vi "ScaledInertialPropertiesToMJ.vi"() -> ()   [LabVIEW 2011]
uses:
  <vilib>/Utility/file.llb/Read From Spreadsheet File (DBL).vi
panel:
  out "pos values":dbl[](array[numeric])
  out "pos":string[](array[string])
  in  "template path":path=path "C:/Users/PPL/Documents/Visual Studio 2015/Projects/Mujoco/mjpro140/RMsimSibelius/5SegRM_template.xml"
  in  "RMsim path":path=path "C:/Users/PPL/Documents/Visual Studio 2015/Projects/Mujoco/mjpro140/RMsim"
  in  "SAVE":bool
  in  "RMsibelius path":path=path "C:/Users/PPL/Documents/Visual Studio 2015/Projects/Mujoco/mjpro140/RMsimSibelius"
  out "mass values":dbl[](array[numeric])
  out "masses":string[](array[string])
  out "length values":dbl[](array[numeric])
  out "lengths":string[](array[string])
  out "radii values":dbl[](array[numeric])
  out "radii":string[](array[string])
  out "MOI values":dbl[](array[numeric])
  out "appended array":string[](array[string])
  in  "indices":dbl[](array[numeric])=[0.0, 2.0, 3.0, 4.0, 5.0]
  in  "file path (dialog if empty)":path
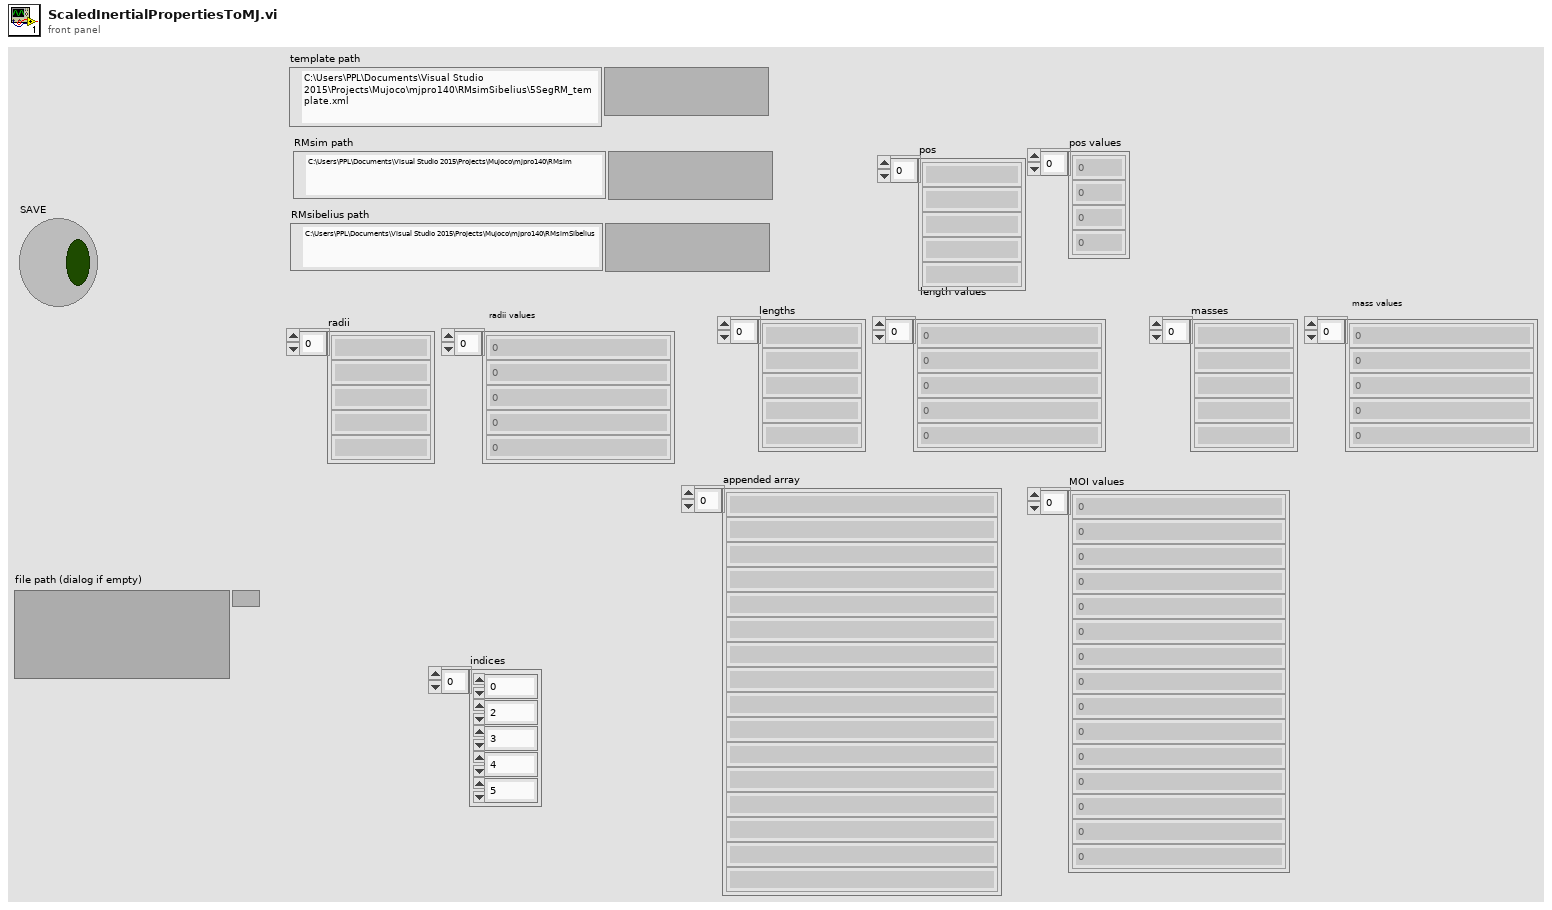
[diagram p1: front panel]
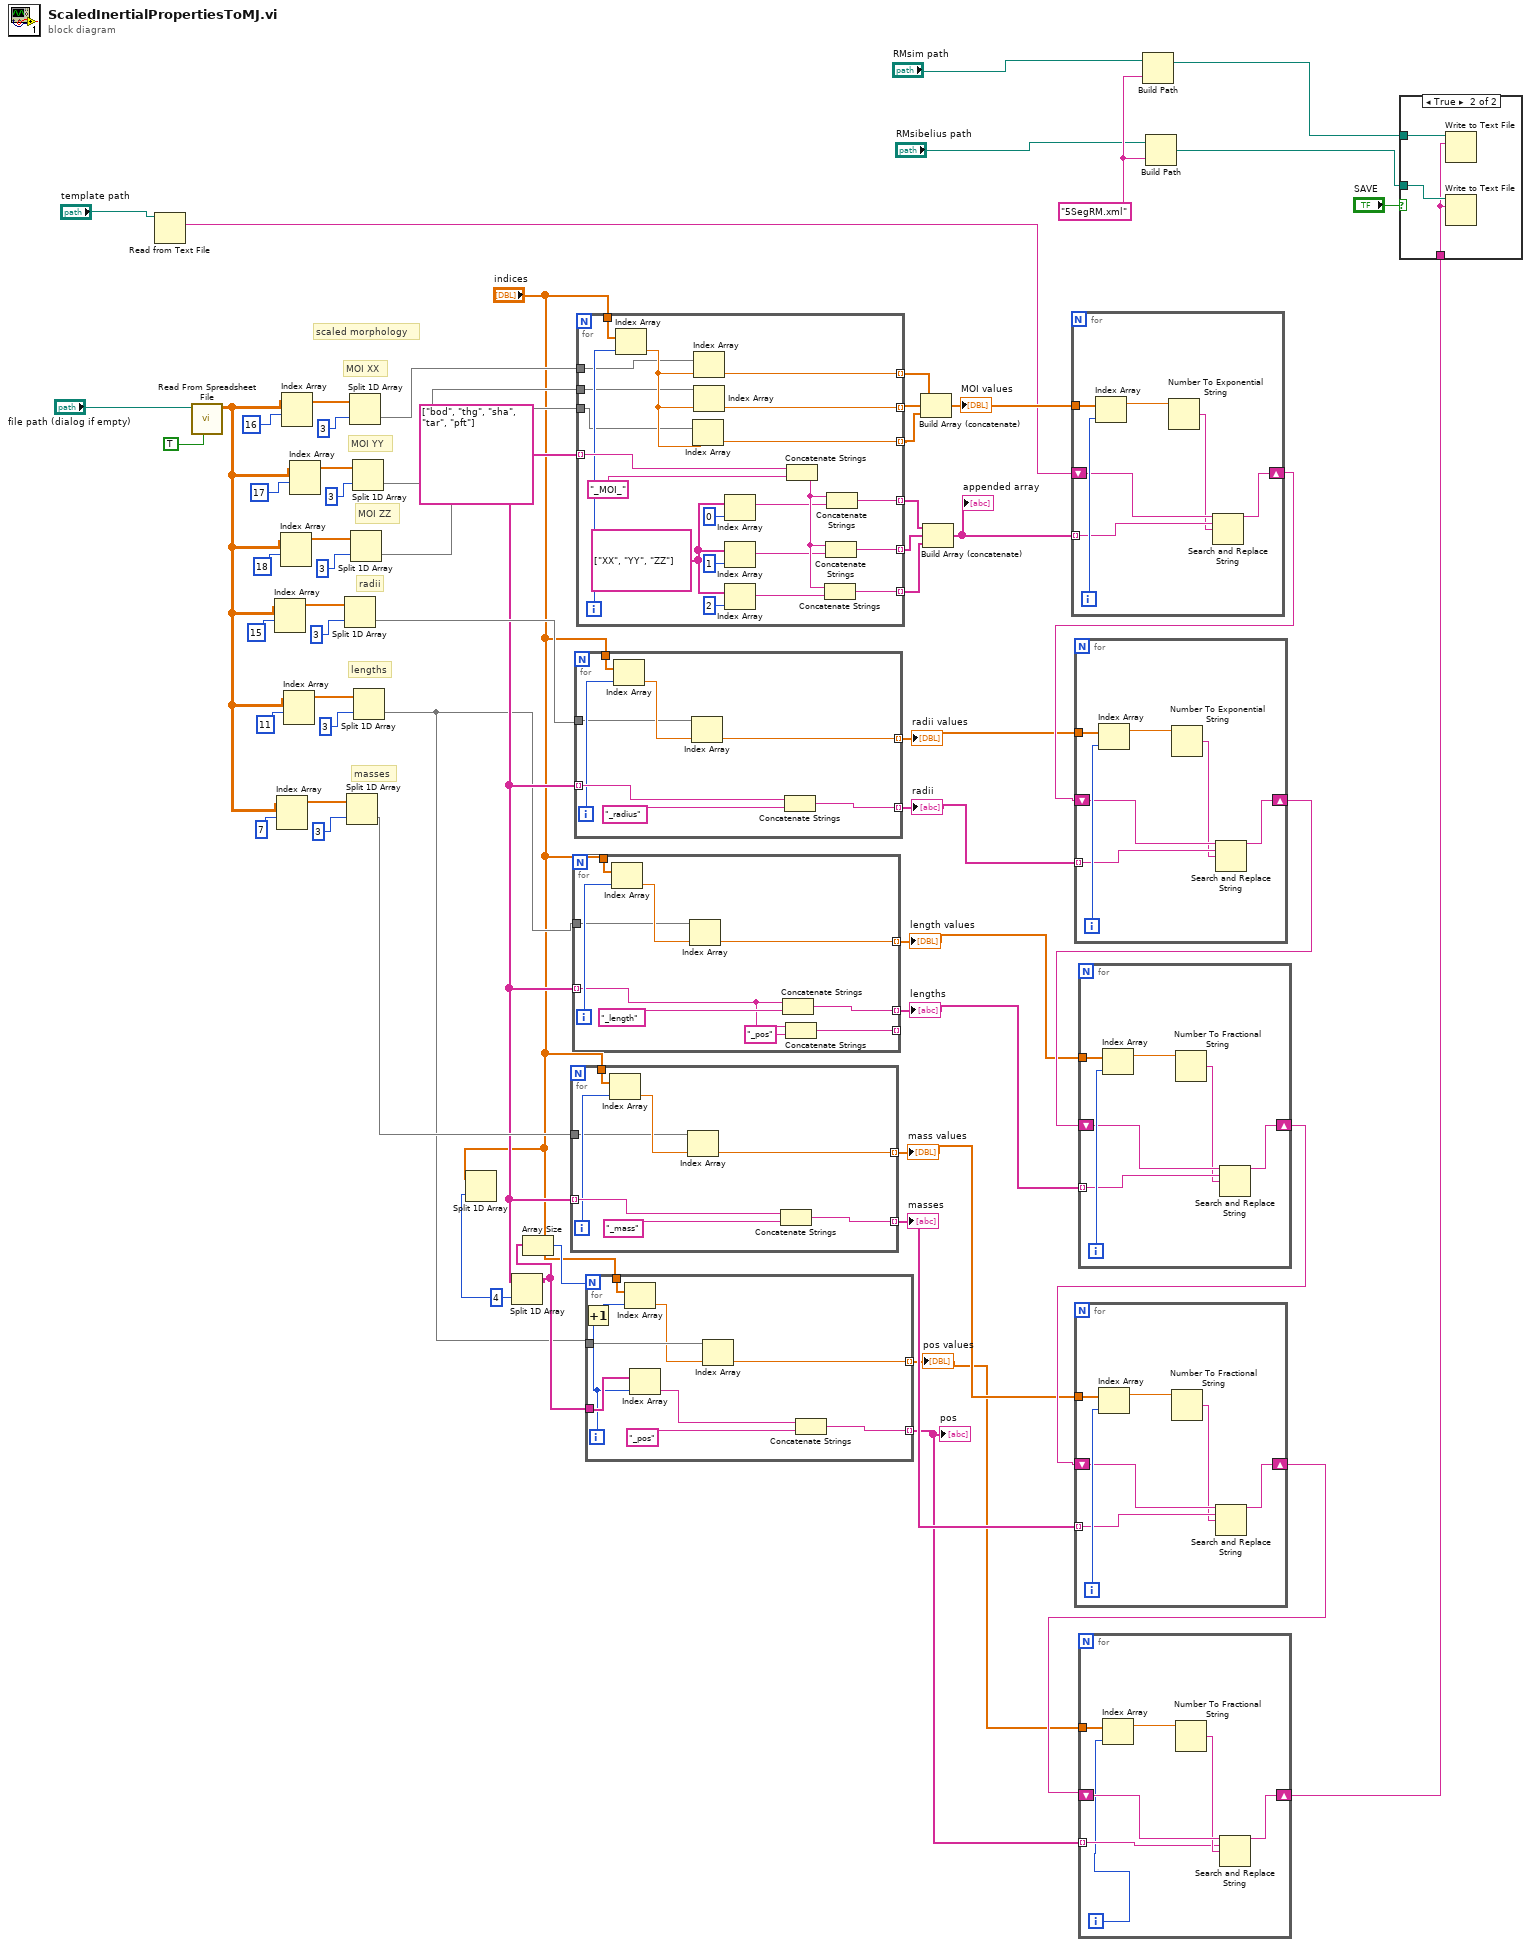
[diagram p0: block diagram]
diagram:
  w4 = 4 ("index")
  w16 = "5SegRM.xml" ("name or relative path")
  w8 = string[] ["bod", "thg", "sha", "tar", "pft"] ("array of strings")
  # "scaled morphology"
  # "lengths"
  # "masses"
  # "radii"
  # "MOI ZZ"
  # "MOI YY"
  # "MOI XX"
  n1 = Read from Text File(file (use dialog)="template path") -> (text=w27:string)  [unwired: 3 in, 3 out]
  n2 = call-poly <vilib>:"Read From Spreadsheet File.vi"("transpose (no:F)"=TRUE, "file path (dialog if empty)"="file path (dialog if empty)") -> ("all rows"=w41:dbl[][])  [unwired: 5 in, 4 out]
  n3 = Index Array(array=w41, index (row)=15) -> (element=w48:dbl[])  [unwired: 1 in]
  n4 = Index Array(array=w41, index (row)=7) -> (element=w42:dbl[])  [unwired: 1 in]
  n5 = Index Array(array=w41, index (row)=18) -> (element=w51:dbl[])  [unwired: 1 in]
  n6 = Index Array(array=w41, index (row)=16) -> (element=w57:dbl[])  [unwired: 1 in]
  n7 = Index Array(array=w41, index (row)=11) -> (element=w45:dbl[])  [unwired: 1 in]
  n8 = Index Array(array=w41, index (row)=17) -> (element=w54:dbl[])  [unwired: 1 in]
  n9 = Split 1D Array(array=w48, index=3) -> (second subarray=w31:dbl[])  [unwired: 1 out]
  n10 = Split 1D Array(array=w42, index=3) -> (second subarray=w30:dbl[])  [unwired: 1 out]
  n11 = Split 1D Array(array=w57, index=3) -> (second subarray=w37:dbl[])  [unwired: 1 out]
  n12 = Split 1D Array(array=w51, index=3) -> (second subarray=w35:dbl[])  [unwired: 1 out]
  n13 = Split 1D Array(array=w54, index=3) -> (second subarray=w36:dbl[])  [unwired: 1 out]
  n14 = Split 1D Array(array=w45, index=3) -> (second subarray=w6:dbl[])  [unwired: 1 out]
  n15 = Split 1D Array(array="indices", index=w4) -> ()  [unwired: 2 out]
  n16 = Split 1D Array(array=w8, index=w4) -> (first subarray=w7:string[])  [unwired: 1 out]
  n17 = Array Size(array=w7) -> (size(s)=w5:i32)
  n18 = for {
    tunnel: w8 -> [w69] mode=indexing
    tunnel: "indices" -> [w67]
    tunnel: w30 -> [w64]
    tunnel: [w63] -> w18 mode=indexing
    tunnel: [w62] -> w19 mode=indexing
    i -> [w66]
    n19 = Index Array(array=w67, index=w66) -> (element=w65:dbl)
    n20 = Index Array(array=w64, index=w65) -> (element=w63:dbl)
    n21 = Concatenate Strings(w69, "_mass" ("string")) -> (w62:string)
  }
  "masses" <- w19
  "mass values" <- w18
  n22 = for {
    tunnel: w8 -> [w72] mode=indexing
    tunnel: "indices" -> [w78]
    tunnel: w6 -> [w75]
    tunnel: [w74] -> w10 mode=indexing
    tunnel: [w73] -> w9 mode=indexing
    tunnel: [w70] -> _ mode=indexing
    i -> [w77]
    n23 = Index Array(array=w78, index=w77) -> (element=w76:dbl)
    n24 = Index Array(array=w75, index=w76) -> (element=w74:dbl)
    n25 = Concatenate Strings(w72, "_length" ("string")) -> (w73:string)
    n26 = Concatenate Strings(w72, "_pos" ("string")) -> (w70:string)
  }
  "lengths" <- w9
  "length values" <- w10
  n27 = for {
    tunnel: w8 -> [w87] mode=indexing
    tunnel: "indices" -> [w85]
    tunnel: w31 -> [w82]
    tunnel: [w81] -> w22 mode=indexing
    tunnel: [w80] -> w23 mode=indexing
    i -> [w84]
    n28 = Index Array(array=w85, index=w84) -> (element=w83:dbl)
    n29 = Index Array(array=w82, index=w83) -> (element=w81:dbl)
    n30 = Concatenate Strings(w87, "_radius" ("string")) -> (w80:string)
  }
  "radii" <- w23
  "radii values" <- w22
  n31 = for {
    tunnel: w8 -> [w109] mode=indexing
    tunnel: [w99] -> w40 mode=indexing
    tunnel: [w98] -> w38 mode=indexing
    tunnel: [w97] -> w39 mode=indexing
    tunnel: "indices" -> [w96]
    tunnel: w37 -> [w93]
    tunnel: w36 -> [w92]
    tunnel: w35 -> [w91]
    tunnel: [w90] -> w34 mode=indexing
    tunnel: [w89] -> w33 mode=indexing
    tunnel: [w88] -> w32 mode=indexing
    i -> [w95]
    w104 = string[] ["XX", "YY", "ZZ"] ("array of strings")
    n32 = Index Array(array=w96, index=w95) -> (element=w94:dbl)
    n33 = Index Array(array=w91, index=w94) -> (element=w88:dbl)
    n34 = Index Array(array=w93, index=w94) -> (element=w90:dbl)
    n35 = Index Array(array=w92, index=w94) -> (element=w89:dbl)
    n36 = Index Array(array=w104, index=0) -> (element=w102:string)
    n37 = Index Array(array=w104, index=1) -> (element=w101:string)
    n38 = Index Array(array=w104, index=2) -> (element=w100:string)
    n39 = Concatenate Strings(w109, "_MOI_" ("string")) -> (w103:string)
    n40 = Concatenate Strings(w103, w100) -> (w97:string)
    n41 = Concatenate Strings(w103, w101) -> (w98:string)
    n42 = Concatenate Strings(w103, w102) -> (w99:string)
  }
  n43 = for {
    N: w5 -> [_]
    tunnel: w7 -> [w113]
    tunnel: "indices" -> [w118]
    tunnel: w6 -> [w117]
    tunnel: [w116] -> w1 mode=indexing
    tunnel: [w115] -> w2 mode=indexing
    i -> [w112]
    n44 = Increment(x=w112) -> (x+1=w110:i32)
    n45 = Index Array(array=w118, index=w110) -> (element=w111:dbl)
    n46 = Index Array(array=w113, index=w112) -> (element=w114:string)
    n47 = Index Array(array=w117, index=w111) -> (element=w116:dbl)
    n48 = Concatenate Strings(w114, "_pos" ("string")) -> (w115:string)
  }
  "pos" <- w2
  "pos values" <- w1
  n49 = Build Array (concatenate)(w34, w33, w32) -> (w28:dbl[])
  "MOI values" <- w28
  n50 = Build Array (concatenate)(w40, w38, w39) -> (w29:string[])
  "appended array" <- w29
  n51 = for {
    tunnel: w29 -> [w124] mode=indexing
    tunnel: w28 -> [w125]
    shift-right: [w122] -> w24
    shift-left: w27 -> [w123]
    i -> [w126]
    n52 = Index Array(array=w125, index=w126) -> (element=w121:dbl)
    n53 = Number To Exponential String(number=w121) -> (E-format string=w120:string)  [unwired: 3 in]
    n54 = Search and Replace String(input string=w123, search string=w124, replace string=w120) -> (result string=w122:string)  [unwired: 5 in, 3 out]
  }
  n55 = for {
    tunnel: w23 -> [w131] mode=indexing
    tunnel: w22 -> [w132]
    shift-right: [w129] -> w21
    shift-left: w24 -> [w130]
    i -> [w133]
    n56 = Index Array(array=w132, index=w133) -> (element=w128:dbl)
    n57 = Number To Exponential String(number=w128) -> (E-format string=w127:string)  [unwired: 3 in]
    n58 = Search and Replace String(input string=w130, search string=w131, replace string=w127) -> (result string=w129:string)  [unwired: 5 in, 3 out]
  }
  n59 = for {
    tunnel: w9 -> [w138] mode=indexing
    tunnel: w10 -> [w139]
    shift-right: [w136] -> w20
    shift-left: w21 -> [w137]
    i -> [w140]
    n60 = Index Array(array=w139, index=w140) -> (element=w135:dbl)
    n61 = Number To Fractional String(number=w135) -> (F-format string=w134:string)  [unwired: 3 in]
    n62 = Search and Replace String(input string=w137, search string=w138, replace string=w134) -> (result string=w136:string)  [unwired: 5 in, 3 out]
  }
  n63 = for {
    tunnel: w19 -> [w145] mode=indexing
    tunnel: w18 -> [w146]
    shift-right: [w143] -> w12
    shift-left: w20 -> [w144]
    i -> [w147]
    n64 = Index Array(array=w146, index=w147) -> (element=w142:dbl)
    n65 = Number To Fractional String(number=w142) -> (F-format string=w141:string)  [unwired: 3 in]
    n66 = Search and Replace String(input string=w144, search string=w145, replace string=w141) -> (result string=w143:string)  [unwired: 5 in, 3 out]
  }
  n67 = for {
    tunnel: w1 -> [w154]
    shift-right: [w152] -> w11
    shift-left: w12 -> [w153]
    tunnel: w2 -> [w149] mode=indexing
    i -> [w148]
    n68 = Index Array(array=w154, index=w148) -> (element=w151:dbl)
    n69 = Number To Fractional String(number=w151) -> (F-format string=w150:string)  [unwired: 3 in]
    n70 = Search and Replace String(input string=w153, search string=w149, replace string=w150) -> (result string=w152:string)  [unwired: 5 in, 3 out]
  }
  n71 = Build Path(base path="RMsim path", name or relative path=w16) -> (appended path=w15:path)
  n72 = Build Path(base path="RMsibelius path", name or relative path=w16) -> (appended path=w25:path)
  n73 = case shown="True" "SAVE" {
    tunnel: w25 -> [_ w157]
    tunnel: w11 -> [_ w156]
    tunnel: w15 -> [_ w155]
    frame False {
    }
    frame True {
      n74 = Write to Text File(file (use dialog)=w155, text=w156) -> ()  [unwired: 2 in, 3 out]
      n75 = Write to Text File(file (use dialog)=w157, text=w156) -> ()  [unwired: 2 in, 3 out]
    }
  }
